vi "Test Composite Image.vi"() -> ()   [LabVIEW 2011]
uses:
  Vec3d Class/Vec3d Class.lvclass
  Take Outline Image.vi
  Gantry Class/Gantry Class.lvclass
  CameraTool Class.lvclass
panel:
  out "Field of View Out":cluster{"x(mm)":dbl, "y(mm)":dbl}
  out "Center":cluster{"X":dbl, "Y":dbl, "Z":dbl}
  in  "Outline Width":dbl
  in  "Config Folder":path=path "C:/Users/husker/Desktop/gantry/Config"
  in  "Field of View":cluster{"Size-X(mm)":dbl, "Size-Y(mm)":dbl}
  in  "Data":cluster{"X":dbl, "Y":dbl, "Z":dbl}
  out "Image":T1(plugin-control)
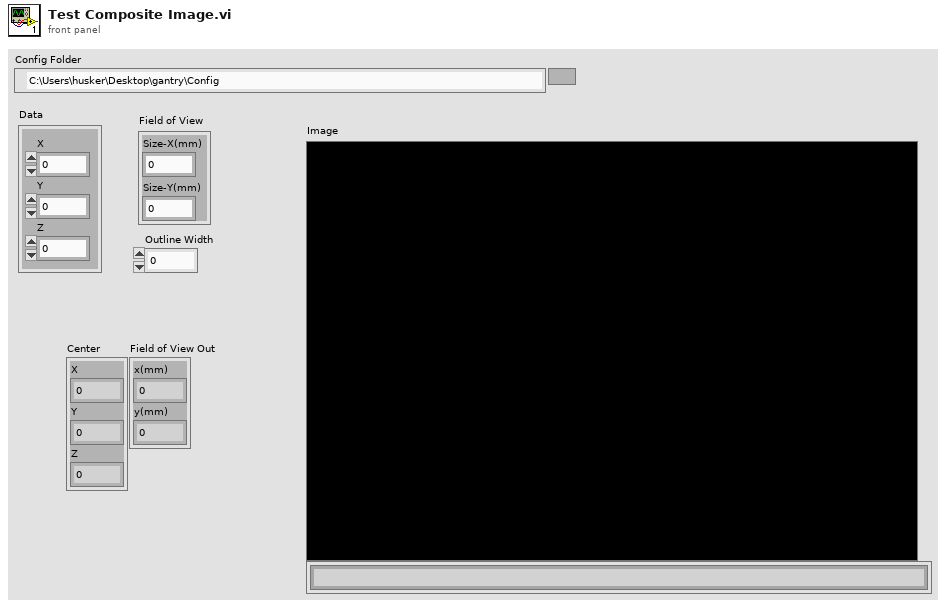
[diagram p1: front panel]
types:
  T1 = typedef "IMAQ Image.ctl" = refnum<image>
  T2 = typedef "Physical Image.ctl" = cluster{"Image Position":refnum<class "Vec3d Class.lvclass">, "Image Reference":T1, "Field of View":cluster{"x(mm)":dbl, "y(mm)":dbl}}
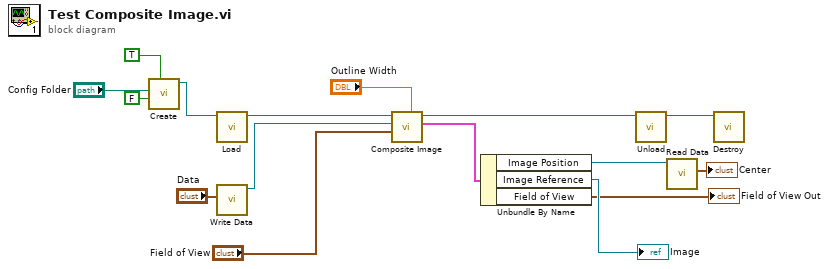
[diagram p0: block diagram]
diagram:
  n1 = call "Create.vi"("Virtual Mode"=TRUE, "HOME?"=FALSE, "Config Folder"="Config Folder") -> ("Gantry out"=w16:refnum<class "Gantry Class.lvclass">)  [unwired: 7 in, 1 out]
  n2 = call "Load.vi"("Gantry In"=w16) -> ("CameraTool out"=w15:refnum<class "CameraTool Class.lvclass">)  [unwired: 9 in, 1 out]
  n3 = call "Write Data.vi"("Data"="Data") -> ("Vec3d Class out"=w11:refnum<class "Vec3d Class.lvclass">)  [unwired: 9 in, 1 out]
  n4 = call-poly "Composite Image.vi"("Outline Width"="Outline Width", "Field of View"="Field of View", "Image Center"=w11, "CameraTool in"=w15) -> ("Physical Image"=w14:T2, "CameraTool out"=w9:refnum<class "CameraTool Class.lvclass">)  [unwired: 5 in, 1 out]
  n5 = Unbundle By Name(w14) -> ("Image Position"=w4:refnum<class "Vec3d Class.lvclass">, "Image Reference"=→"Image":T1, "Field of View"=→"Field of View Out":cluster{"x(mm)":dbl, "y(mm)":dbl})
  n6 = call "Unload.vi"("CameraTool in"=w9) -> ("Gantry out"=w8:refnum<class "Gantry Class.lvclass">)  [unwired: 9 in, 1 out]
  n7 = call-dynamic "Read Data.vi"("Vec3d Class in"=w4) -> ("Data"=→"Center":cluster{"X":dbl, "Y":dbl, "Z":dbl})  [unwired: 8 in, 2 out]
  n8 = call "Destroy.vi"("Gantry Class in"=w8) -> ()  [unwired: 10 in, 1 out]
